vi "GVSDV Get Control Value.vi"(6 "nData":i32, 8 "sData":string="Basic", 9 "sControlName":string="Basic", 10 "pVIRef":refnum<vi>, 11 "sAction":string="Basic") -> (0 "Boolen":bool, 1 "String":string="Basic", 2 "Numeric":i32, 3 "pSPRef":refnum<vi>, 4 "bResult":bool)   [LabVIEW 2013]
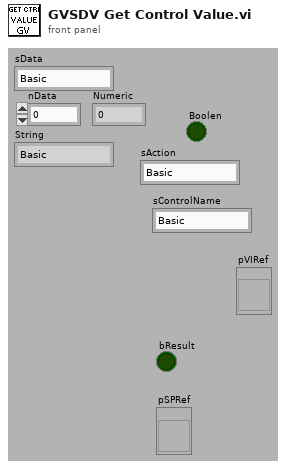
[diagram p1: front panel]
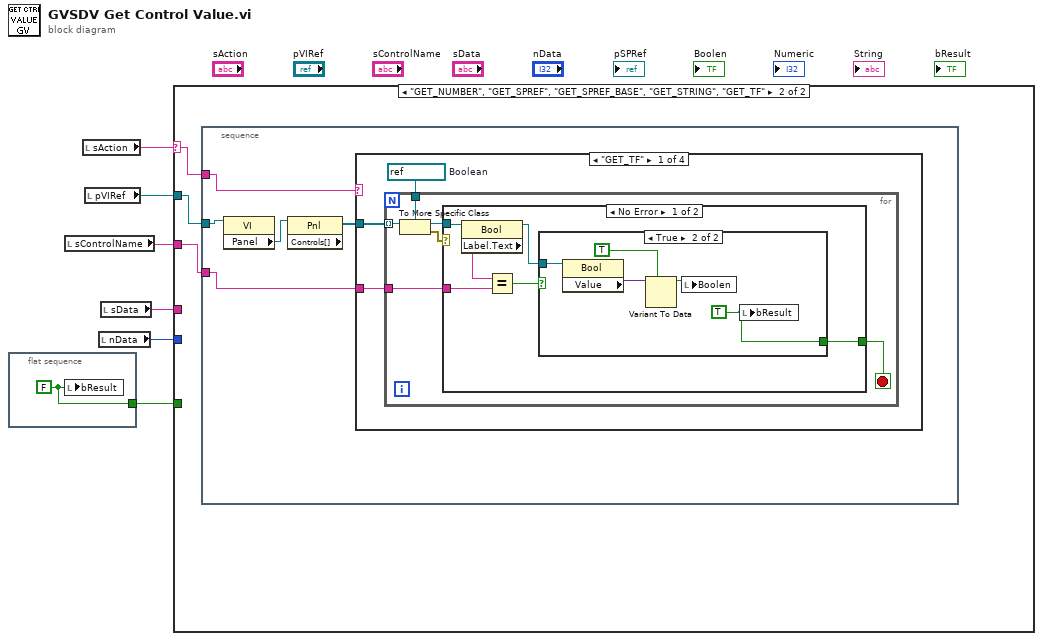
[diagram p0: block diagram]
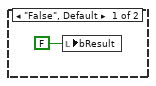
[diagram p2: hidden frame]
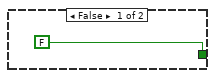
[diagram p3: hidden frame]
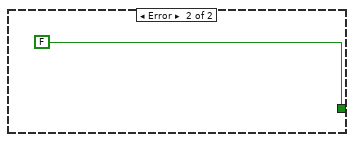
[diagram p4: hidden frame]
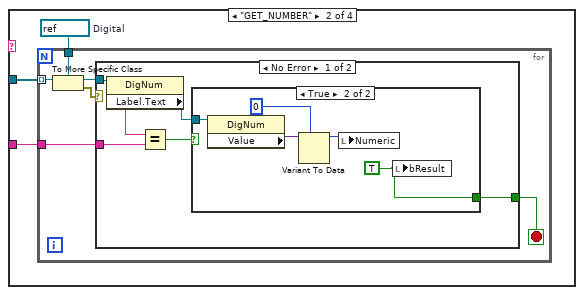
[diagram p5: hidden frame]
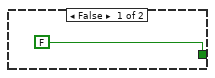
[diagram p6: hidden frame]
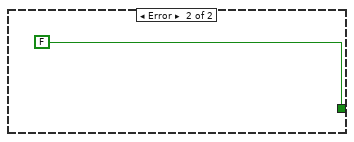
[diagram p7: hidden frame]
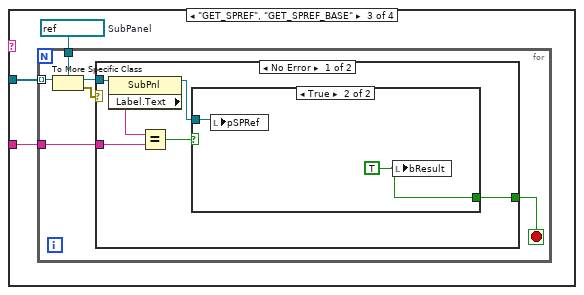
[diagram p8: hidden frame]
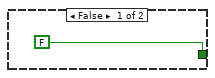
[diagram p9: hidden frame]
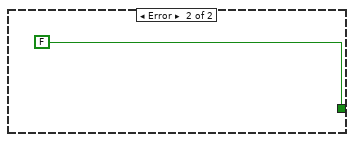
[diagram p10: hidden frame]
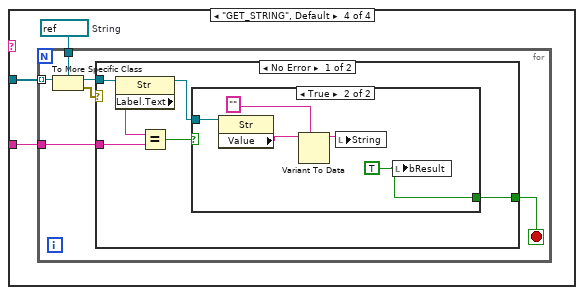
[diagram p11: hidden frame]
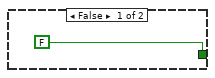
[diagram p12: hidden frame]
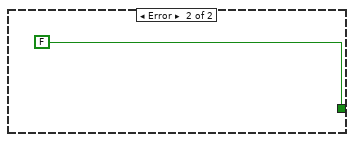
[diagram p13: hidden frame]
diagram:
  n1 = flat-sequence {
    tunnel: [w7] -> w1
    frame #0 {
      w7 = FALSE ("bResult")
      n2 = local write "bResult"(w7) -> ()
    }
  }
  n3 = local read "sControlName"() -> (w4:string)
  n4 = local read "sAction"() -> (w5:string)
  n5 = local read "pVIRef"() -> (w6:refnum<vi>)
  n6 = local read "nData"() -> (w2:i32)
  n7 = local read "sData"() -> (w3:string)
  n8 = case shown="\"GET_NUMBER\", \"GET_SPREF\", \"GET_SPREF_BASE\", \"GET_STRING\", \"GET_TF\"" w5 {
    selector: w5 -> [_ w10]
    tunnel: w4 -> [_ w9]
    tunnel: w6 -> [_ w11]
    tunnel: w3 -> [_ _]
    tunnel: w2 -> [_ _]
    tunnel: w1 -> [_ _]
    frame "False", Default {
      n9 = local write "bResult"(FALSE ("bResult")) -> ()
    }
    frame "GET_NUMBER", "GET_SPREF", "GET_SPREF_BASE", "GET_STRING", "GET_TF" {
      n10 = stacked-sequence {
        tunnel: w11 -> [w16]
        tunnel: w10 -> [w13]
        tunnel: w9 -> [w12]
        frame #0 {
          n11 = property class="VI"(reference=w16) -> ("Panel"=w15:refnum<vi>)  [unwired: 1 in, 2 out]
          n12 = property class="Pnl"(reference=w15) -> ("Controls[]"=w14:refnum<vi>[])  [unwired: 1 in, 2 out]
          n13 = case shown="\"GET_TF\"" w13 {
            tunnel: w14 -> [w18 w40 w62 w81]
            tunnel: w12 -> [w17 w39 w61 w80]
            frame "GET_TF" {
              w19 = refnum<vi> refnum  # Boolean
              n14 = for {
                tunnel: w18 -> [w25] mode=indexing
                tunnel: w19 -> [w24]
                tunnel: w17 -> [w20]
                stop <- w21 stop-if-true
                n15 = To More Specific Class(target class=w24, reference=w25) -> (specific class reference=w22:refnum<vi>, error out=w23:errorcluster)  [unwired: 1 in]
                n16 = case shown="No Error" w23 {
                  tunnel: w22 -> [w28 _]
                  tunnel: [w31 FALSE] -> w21
                  tunnel: w20 -> [w29 _]
                  frame No Error {
                    n17 = property class="Bool"(reference=w28) -> (reference out=w27:refnum<vi>, "Label.Text"=w26:string)  [unwired: 1 in, 1 out]
                    n18 = Equal?(x=w26, y=w29) -> (x = y?=w30:bool)
                    n19 = case shown="True" w30 {
                      tunnel: [FALSE w33] -> w31
                      tunnel: w27 -> [_ w37]
                      frame False {
                      }
                      frame True {
                        w33 = TRUE ("bResult")
                        n20 = property class="Bool"(reference=w37) -> ("Value"=w36:variant)  [unwired: 1 in, 2 out]
                        n21 = Variant To Data(type=TRUE, Variant=w36) -> (data=w34:bool)  [unwired: 1 in, 1 out]
                        n22 = local write "Boolen"(w34) -> ()
                        n23 = local write "bResult"(w33) -> ()
                      }
                    }
                  }
                  frame Error {
                  }
                }
              }
            }
            frame "GET_NUMBER" {
              w41 = refnum<vi> refnum  # Digital
              n24 = for {
                tunnel: w40 -> [w47] mode=indexing
                tunnel: w41 -> [w46]
                tunnel: w39 -> [w42]
                stop <- w43 stop-if-true
                n25 = To More Specific Class(target class=w46, reference=w47) -> (specific class reference=w44:refnum<vi>, error out=w45:errorcluster)  [unwired: 1 in]
                n26 = case shown="No Error" w45 {
                  tunnel: w44 -> [w50 _]
                  tunnel: [w53 FALSE] -> w43
                  tunnel: w42 -> [w51 _]
                  frame No Error {
                    n27 = property class="DigNum"(reference=w50) -> (reference out=w49:refnum<vi>, "Label.Text"=w48:string)  [unwired: 1 in, 1 out]
                    n28 = Equal?(x=w48, y=w51) -> (x = y?=w52:bool)
                    n29 = case shown="True" w52 {
                      tunnel: [FALSE w57] -> w53
                      tunnel: w49 -> [_ w59]
                      frame False {
                      }
                      frame True {
                        w57 = TRUE ("bResult")
                        n30 = property class="DigNum"(reference=w59) -> ("Value"=w58:variant)  [unwired: 1 in, 2 out]
                        n31 = Variant To Data(type=0 ("Numeric"), Variant=w58) -> (data=w55:i32)  [unwired: 1 in, 1 out]
                        n32 = local write "Numeric"(w55) -> ()
                        n33 = local write "bResult"(w57) -> ()
                      }
                    }
                  }
                  frame Error {
                  }
                }
              }
            }
            frame "GET_SPREF", "GET_SPREF_BASE" {
              w63 = refnum<vi> refnum  # SubPanel
              n34 = for {
                tunnel: w62 -> [w69] mode=indexing
                tunnel: w63 -> [w68]
                tunnel: w61 -> [w64]
                stop <- w65 stop-if-true
                n35 = To More Specific Class(target class=w68, reference=w69) -> (specific class reference=w66:refnum<vi>, error out=w67:errorcluster)  [unwired: 1 in]
                n36 = case shown="No Error" w67 {
                  tunnel: w66 -> [w72 _]
                  tunnel: [w75 FALSE] -> w65
                  tunnel: w64 -> [w73 _]
                  frame No Error {
                    n37 = property class="SubPnl"(reference=w72) -> (reference out=w71:refnum<vi>, "Label.Text"=w70:string)  [unwired: 1 in, 1 out]
                    n38 = Equal?(x=w70, y=w73) -> (x = y?=w74:bool)
                    n39 = case shown="True" w74 {
                      tunnel: [FALSE w78] -> w75
                      tunnel: w71 -> [_ w77]
                      frame False {
                      }
                      frame True {
                        w78 = TRUE ("bResult")
                        n40 = local write "pSPRef"(w77) -> ()
                        n41 = local write "bResult"(w78) -> ()
                      }
                    }
                  }
                  frame Error {
                  }
                }
              }
            }
            frame "GET_STRING", Default {
              w82 = refnum<vi> refnum  # String
              n42 = for {
                tunnel: w81 -> [w88] mode=indexing
                tunnel: w82 -> [w87]
                tunnel: w80 -> [w83]
                stop <- w84 stop-if-true
                n43 = To More Specific Class(target class=w87, reference=w88) -> (specific class reference=w85:refnum<vi>, error out=w86:errorcluster)  [unwired: 1 in]
                n44 = case shown="No Error" w86 {
                  tunnel: w85 -> [w91 _]
                  tunnel: [w94 FALSE] -> w84
                  tunnel: w83 -> [w92 _]
                  frame No Error {
                    n45 = property class="Str"(reference=w91) -> (reference out=w90:refnum<vi>, "Label.Text"=w89:string)  [unwired: 1 in, 1 out]
                    n46 = Equal?(x=w89, y=w92) -> (x = y?=w93:bool)
                    n47 = case shown="True" w93 {
                      tunnel: [FALSE w98] -> w94
                      tunnel: w90 -> [_ w100]
                      frame False {
                      }
                      frame True {
                        w98 = TRUE ("bResult")
                        n48 = property class="Str"(reference=w100) -> ("Value"=w99:string)  [unwired: 1 in, 2 out]
                        n49 = Variant To Data(type="" ("String"), Variant=w99) -> (data=w96:string)  [unwired: 1 in, 1 out]
                        n50 = local write "String"(w96) -> ()
                        n51 = local write "bResult"(w98) -> ()
                      }
                    }
                  }
                  frame Error {
                  }
                }
              }
            }
          }
        }
      }
    }
  }
